vi "terminal_display_handler.vi"(0 "actions (write=def)":T1=enum."write", 2 "terminal_name (in)":string, 3 "line in":string, 5 "error in (no error)":errorcluster, 6 "terminal_ref (in)":refnum<vi>, 8 "buffer (in)":i32) -> (19 "error out":errorcluster)   [LabVIEW 2016]
uses:
  controls/terminal_display_handler_actions.ctl
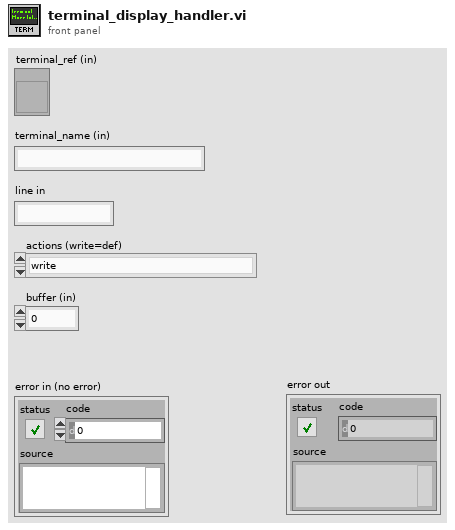
[diagram p1: front panel]
types:
  T1 = typedef "terminal_display_handler_actions.ctl" = enum16{"clear", "clear_all", "init", "reset", "write"}
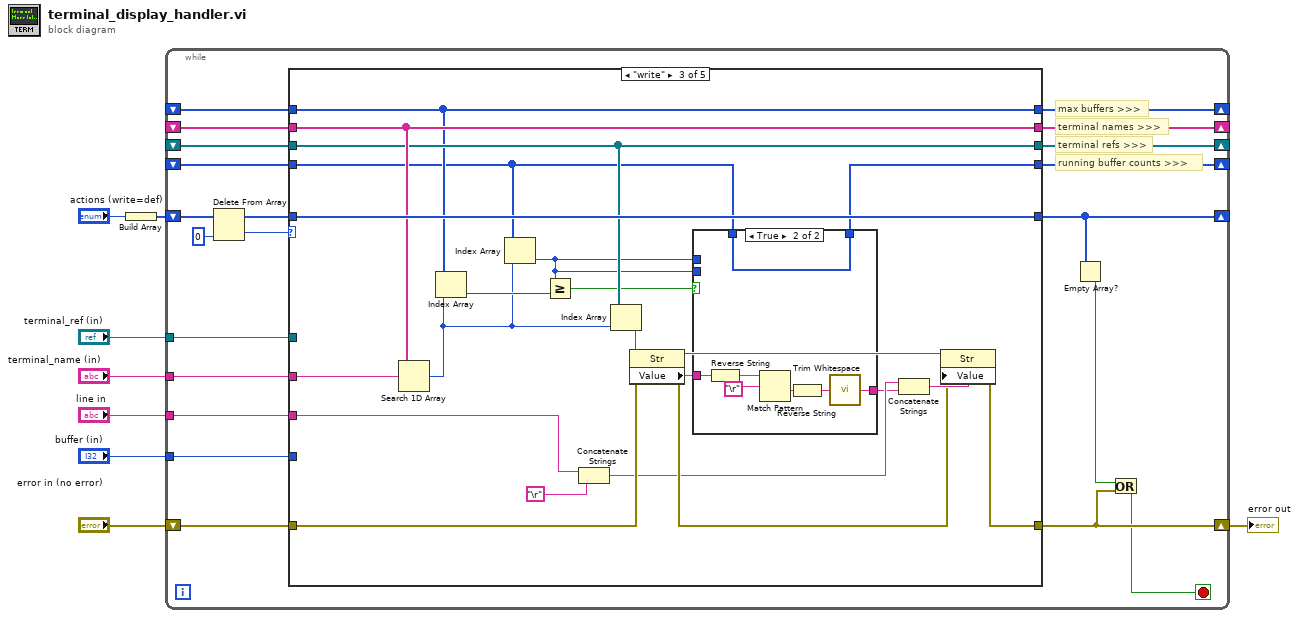
[diagram p0: block diagram]
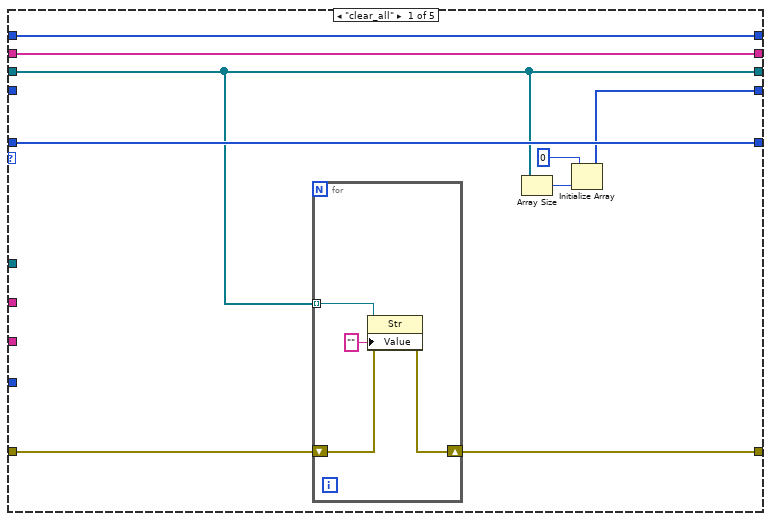
[diagram p2: hidden frame]
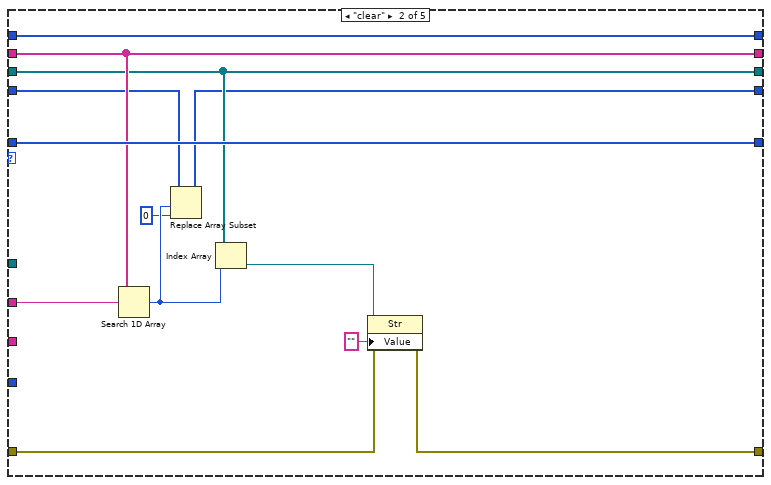
[diagram p3: hidden frame]
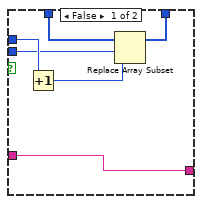
[diagram p4: hidden frame]
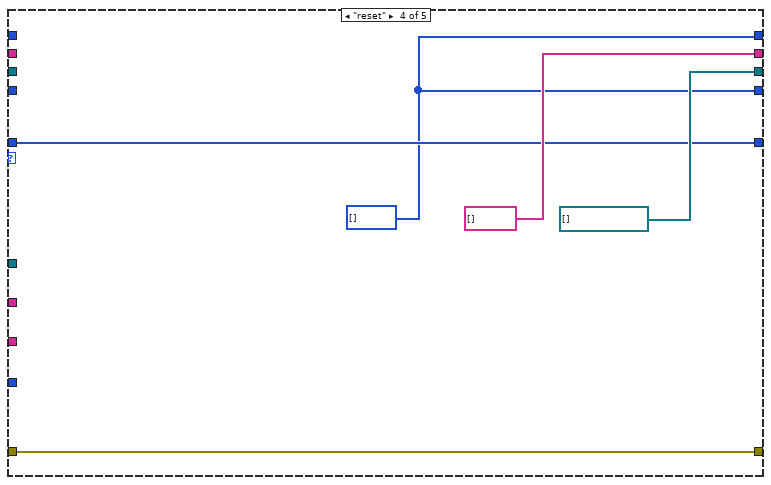
[diagram p5: hidden frame]
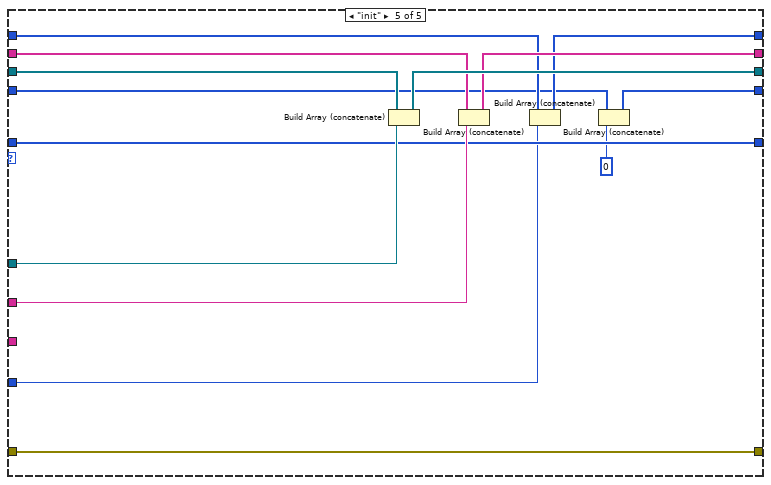
[diagram p6: hidden frame]
diagram:
  n1 = Build Array("actions (write=def)") -> (w7:T1[])
  n2 = while {
    shift-right: [w14] -> _
    shift-left: w7 -> [w29]
    shift-right: [w23] -> _
    shift-left: _ -> [w25]
    shift-right: [w20] -> _
    shift-left: _ -> [w22]
    tunnel: "terminal_ref (in)" -> [w24]
    tunnel: "terminal_name (in)" -> [w21]
    shift-right: [w17] -> _
    shift-left: _ -> [w18]
    tunnel: "buffer (in)" -> [w19]
    shift-right: [w12] -> w1
    shift-left: "error in (no error)" -> [w16]
    tunnel: "line in" -> [w15]
    shift-right: [w9] -> _
    shift-left: _ -> [w10]
    stop <- w11 stop-if-true
    # "running buffer counts >>>"
    # "terminal refs >>>"
    # "terminal names >>>"
    # "max buffers >>>"
    n3 = Delete From Array(array=w29, index=0) -> (deleted portion=w27:T1, array with subset deleted=w26:T1[])  [unwired: 1 in]
    n4 = case shown="\"write\"" w27 {
      tunnel: w26 -> [w38 w55 w77 w93 w103]
      tunnel: [w38 w55 w77 w93 w103] -> w14
      tunnel: w25 -> [w33 w49 w73 _ w109]
      tunnel: w24 -> [_ _ _ _ w108]
      tunnel: [w33 w49 w73 refnum<vi>[] [] w107] -> w23
      tunnel: w22 -> [w36 w51 w75 _ w106]
      tunnel: w21 -> [_ w50 w74 _ w105]
      tunnel: [w36 w51 w75 string[] [] w104] -> w20
      tunnel: w19 -> [_ _ _ _ w102]
      tunnel: w18 -> [w37 w54 w70 _ w101]
      tunnel: [w37 w54 w70 w91 w100] -> w17
      tunnel: w16 -> [w35 w53 w76 w92 w96]
      tunnel: [w34 w47 w64 w92 w96] -> w12
      tunnel: w15 -> [_ _ w71 _ _]
      tunnel: w10 -> [_ w46 w61 _ w99]
      tunnel: [w30 w43 w60 w91 w98] -> w9
      frame "clear_all" {
        n5 = for {
          tunnel: w33 -> [w42] mode=indexing
          shift-right: [w39] -> w34
          shift-left: w35 -> [w40]
          n6 = property class="Str"(reference=w42, error in=w40, "Value"="") -> (error out=w39:errorcluster)  [unwired: 1 out]
        }
        n7 = Array Size(array=w33) -> (size(s)=w32:i32)
        n8 = Initialize Array(0, w32) -> (w30:i32[])
      }
      frame "clear" {
        n9 = Search 1D Array(1D array=w51, element=w50) -> (index of element=w45:i32)  [unwired: 1 in]
        n10 = Replace Array Subset(array=w46, new element=0 ("new element/subarray"), index=w45) -> (w43:i32[])
        n11 = Index Array(array=w49, index=w45) -> (element=w48:refnum<vi>)
        n12 = property class="Str"(reference=w48, error in=w53, "Value"="") -> (error out=w47:errorcluster)  [unwired: 1 out]
      }
      frame "write" {
        n13 = Search 1D Array(1D array=w75, element=w74) -> (index of element=w59:i32)  [unwired: 1 in]
        n14 = Index Array(array=w70, index=w59) -> (element=w69:i32)
        n15 = Index Array(array=w61, index=w59) -> (element=w58:i32)
        n16 = Greater Or Equal?(x=w58, y=w69) -> (x >= y?=w66:bool)
        n17 = Concatenate Strings(w71, "\r") -> (w57:string)
        n18 = Index Array(array=w73, index=w59) -> (element=w72:refnum<vi>)
        n19 = property class="Str"(reference=w72, error in=w76) -> (reference out=w63:refnum<vi>, error out=w62:errorcluster, "Value"=w68:string)
        n20 = case shown="True" w66 {
          tunnel: w68 -> [w83 w90]
          tunnel: [w83 w88] -> w56
          tunnel: w61 -> [w81 w86]
          tunnel: [w78 w86] -> w60
          tunnel: w58 -> [w82 _]
          tunnel: w58 -> [w79 _]
          frame False {
            n21 = Increment(x=w82) -> (x+1=w80:i32)
            n22 = Replace Array Subset(array=w81, new element=w80, index=w79) -> (w78:i32[])
          }
          frame True {
            n23 = Reverse String(1:w90) -> (0:w85:string)
            n24 = Match Pattern(string=w85, regular expression="\r") -> (after substring=w89:string)  [unwired: 1 in, 3 out]
            n25 = Reverse String(1:w89) -> (0:w84:string)
            n26 = call <vilib>:"Trim Whitespace.vi"("string"=w84) -> ("trimmed string"=w88:string)  [unwired: 1 in]
          }
        }
        n27 = Concatenate Strings(w57, w56) -> (w65:string)
        n28 = property class="Str"(reference=w63, error in=w62, "Value"=w65) -> (error out=w64:errorcluster)  [unwired: 1 out]
      }
      frame "reset" {
        w91 = i32[] []
      }
      frame "init" {
        n29 = Build Array (concatenate)(w109, w108) -> (w107:refnum<vi>[])
        n30 = Build Array (concatenate)(w106, w105) -> (w104:string[])
        n31 = Build Array (concatenate)(w101, w102) -> (w100:i32[])
        n32 = Build Array (concatenate)(w99, 0) -> (w98:i32[])
      }
    }
    n33 = Empty Array?(array=w14) -> (empty?=w13:bool)
    n34 = Or(x=w13, y=w12) -> (x .or. y?=w11:bool)
  }
  "error out" <- w1
